vi "Periodic Tasks.vi"(8 "error in":errorcluster) -> ()   [LabVIEW 2020]
doc: "This VI runs in parallel to other tasks. It can contain as many user-defined periodic loops as you need. These can carry out PID or other sorts of timed response."
uses:
  <vilib>/Rock Robotics/WPI/ThirdParty/Phoenix-LabVIEW/Motor Controller/Controls/CTRE_Phoenix_MotorControl_ControlMode.ctl
  V1_nauru_2023_06_22/Global 1.vi
  <vilib>/Rock Robotics/Network Tables/NT Read Number.vi
  <vilib>/Rock Robotics/Network Tables/NT Write Number.vi
  <vilib>/Rock Robotics/WPI/Utilities/WPI_GetSetVariantRefNum.vi
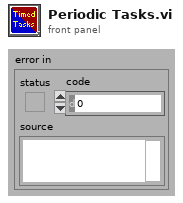
[diagram p1: front panel]
types:
  T1 = typedef "CTRE_Phoenix_MotorControl_ControlMode.ctl" = u16
  T2 = typedef "WPI_SwitchDevRef.ctl" = cluster{"DevStatus":errorcluster, "DIO Channel":T3, "CntIndex":T4, "Normally Closed":bool}
  T3 = typedef "FPGA_DIOChannel.ctl" = enum8{"DIO 0", "DIO 1", "DIO 2", "DIO 3", "DIO 4", "DIO 5", "DIO 6", "DIO 7", "DIO 8", "DIO 9", "DIO MXP 0", "DIO MXP 1", "DIO MXP 2", "DIO MXP 3", "DIO MXP 4", "DIO MXP 5", "DIO MXP 6", "DIO MXP 7", "DIO MXP 8", "DIO MXP 9", "DIO MXP 10", "DIO MXP 11", "DIO MXP 12", "DIO MXP 13", "DIO MXP 14", "DIO MXP 15", "SPI Port CS1", "SPI Port CS2", "SPI Port CS3", "SPI Port MISO", "SPI Port MOSI", "Invalid"}
  T4 = typedef "FPGA_CounterCtrSystemIndex.ctl" = enum8{"Ctr 0", "Ctr 1", "Ctr 2", "Ctr 3", "Ctr 4", "Ctr 5", "Ctr 6", "Ctr 7", "Invalid"}
  T5 = cluster{"Yaw":dbl, "Roll":dbl, "Pitch":dbl, "Heading":dbl, "Fused Heading":dbl}
  T6 = typedef "WPI_MotorControlDeviceRef.ctl" = cluster{"DeviceStatus":errorcluster, "Type":T7, "PWM":cluster{"PWM Channel":T8, "DeadBand":T9}, "CAN":cluster{"Device Number":u8, "SetOutput VI Ref":variant, "GetOutput VI Ref":variant, "Enable VI Ref":variant, "Disable VI Ref":variant, "Data":variant}, "Invert":bool, "DIO PWM":cluster{"PWM \"Enable\" Channel":T8, "DIOChannel":T3, "PWM Rate":dbl}}
  T7 = typedef "WPI_MotorControlType.ctl" = enum16{"PWM", "CAN", "DIO PWM"}
  T8 = typedef "FPGA_DIOPWMChannel.ctl" = enum8{"PWM 0", "PWM 1", "PWM 2", "PWM 3", "PWM 4", "PWM 5", "PWM 6", "PWM 7", "PWM 8", "PWM 9", "PWM MXP 0", "PWM MXP 1", "PWM MXP 2", "PWM MXP 3", "PWM MXP 4", "PWM MXP 5", "PWM MXP 6", "PWM MXP 7", "PWM MXP 8", "PWM MXP 9", "Invalid"}
  T9 = typedef "WPI_PWMDeadband.ctl" = cluster{"Name":string, "maxPositivePwm":i32, "minPositivePwm":i32, "centerPwm":i32, "maxNegativePwm":i32, "minNegativePwm":i32, "angularRange":u16}
  T10 = typedef "WPI_RobotDriveDevRef.ctl" = cluster{"DevStatus":errorcluster, "Motors[]":T6[], "Square Inputs":bool, "Max Output":dbl}
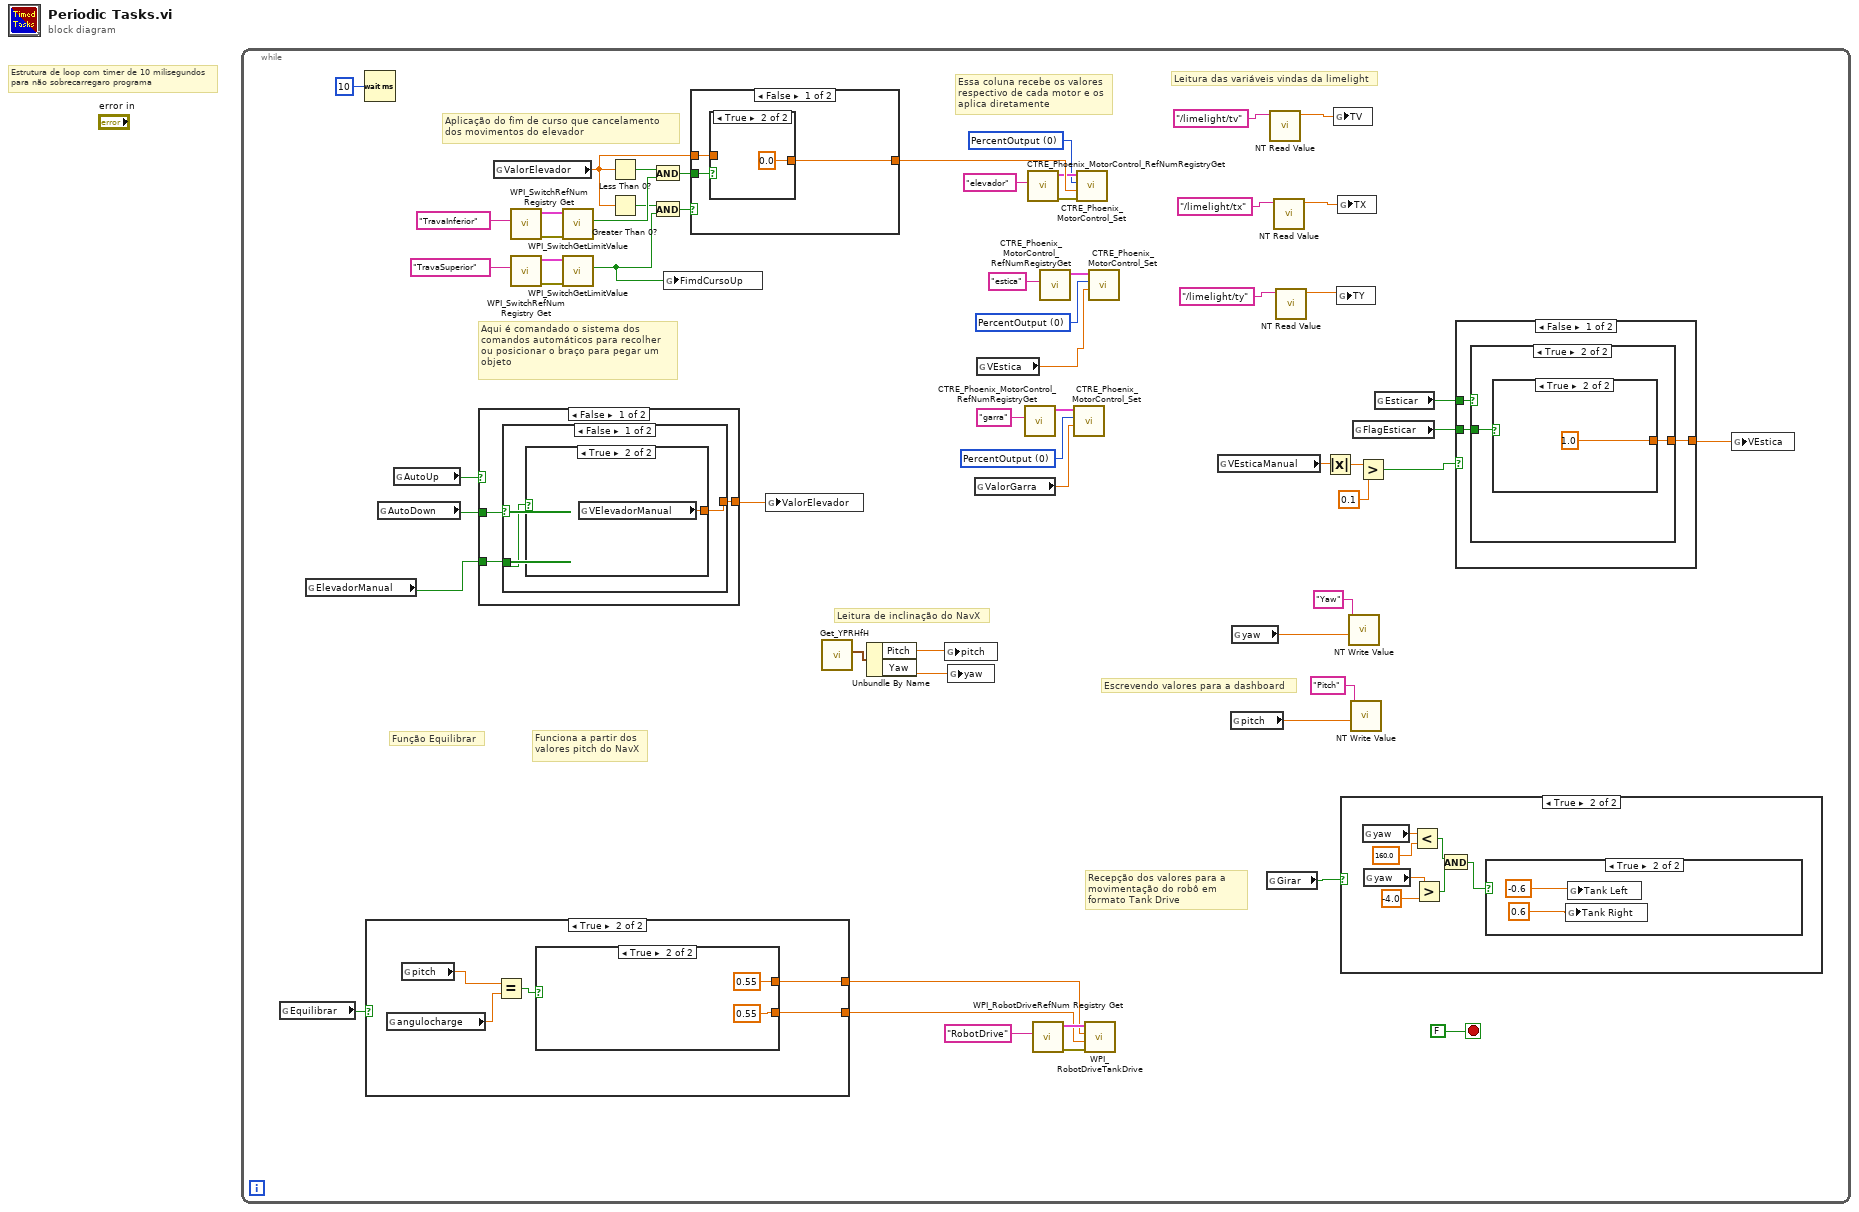
[diagram p0: block diagram]
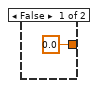
[diagram p2: hidden frame]
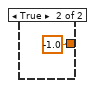
[diagram p3: hidden frame]
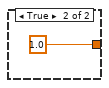
[diagram p4: hidden frame]
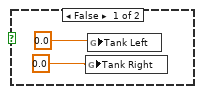
[diagram p6: hidden frame]
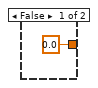
[diagram p7: hidden frame]
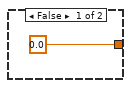
[diagram p8: hidden frame]
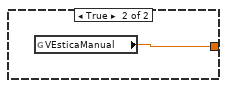
[diagram p9: hidden frame]
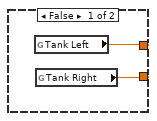
[diagram p10: hidden frame]
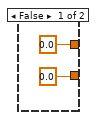
[diagram p11: hidden frame]
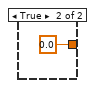
[diagram p13: hidden frame]
diagram:
  # "Estrutura de loop com timer de 10 milisegundos para não sobrecarregaro programa"
  n1 = while {
    stop <- FALSE stop-if-true
    w14 = T1 0 items=["PercentOutput"=0, "Position"=1, "Velocity"=2, "Current"=3, "Follower"=5, "MotionProfile"=6, "MotionMagic"=7, "MotionProfileArc"=10, "Disabled"=15] ("Control Mode")
    w36 = T1 0 items=["PercentOutput"=0, "Position"=1, "Velocity"=2, "Current"=3, "Follower"=5, "MotionProfile"=6, "MotionMagic"=7, "MotionProfileArc"=10, "Disabled"=15] ("Control Mode")
    w50 = T1 0 items=["PercentOutput"=0, "Position"=1, "Velocity"=2, "Current"=3, "Follower"=5, "MotionProfile"=6, "MotionMagic"=7, "MotionProfileArc"=10, "Disabled"=15] ("Control Mode")
    # "Escrevendo valores para a dashboard"
    # "Funciona a partir dos valores pitch do NavX"
    # "Função Equilibrar"
    # "Leitura de inclinação do NavX"
    # "Leitura das variáveis vindas da limelight"
    # "Recepção dos valores para a movimentação do robô em formato Tank Drive"
    # "Aplicação do fim de curso que cancelamento dos movimentos do elevador"
    # "Aqui é comandado o sistema dos comandos automáticos para recolher ou posicionar o braço para pegar um objeto"
    # "Essa coluna recebe os valores\nrespectivo de cada motor e os\naplica diretamente"
    n2 = global read "Global 1.vi" "Equilibrar"() -> (w27:bool)
    n3 = global read "Global 1.vi" "ElevadorManual"() -> (w2:bool)
    n4 = Wait (ms)(milliseconds to wait=u32 10) -> ()  [unwired: 1 out]
    n5 = case shown="True" w27 {
      tunnel: [w90 w91] -> w25
      tunnel: [w89 w92] -> w24
      frame False {
        n6 = global read "Global 1.vi" "Tank Left"() -> (w90:dbl)
        n7 = global read "Global 1.vi" "Tank Right"() -> (w89:dbl)
      }
      frame True {
        n8 = global read "Global 1.vi" "angulocharge"() -> (w94:dbl)
        n9 = global read "Global 1.vi" "pitch"() -> (w95:dbl)
        n10 = Equal?(x=w95, y=w94) -> (x = y?=w93:bool)
        n11 = case shown="True" w93 {
          tunnel: [0.0 ("Tank Right") 0.55 ("Tank Right")] -> w92
          tunnel: [0.0 ("Tank Left") 0.55 ("Tank Left")] -> w91
          frame False {
          }
          frame True {
          }
        }
      }
    }
    n12 = global read "Global 1.vi" "AutoDown"() -> (w3:bool)
    n13 = global read "Global 1.vi" "AutoUp"() -> (w4:bool)
    n14 = case shown="False" w4 {
      tunnel: w3 -> [w62 _]
      tunnel: [w61 1.0] -> w1
      tunnel: w2 -> [w60 _]
      frame False {
        n15 = case shown="False" w62 {
          tunnel: [w63 -1.0] -> w61
          tunnel: w60 -> [w64 _]
          frame False {
            n16 = case shown="True" w64 {
              tunnel: [0.0 ("ValorElevador") w66] -> w63
              frame False {
              }
              frame True {
                n17 = global read "Global 1.vi" "VElevadorManual"() -> (w66:dbl)
              }
            }
          }
          frame True {
          }
        }
      }
      frame True {
      }
    }
    n18 = global read "Global 1.vi" "ValorElevador"() -> (w39:dbl)
    n19 = call <vilib>:"WPI_SwitchRefNum Registry Get.vi"("refnum name"="TravaInferior") -> ("error out"=w46:errorcluster, "SwitchDevRef"=w45:T2)  [unwired: 9 in]
    n20 = call <vilib>:"WPI_SwitchRefNum Registry Get.vi"("refnum name"="TravaSuperior") -> ("error out"=w49:errorcluster, "SwitchDevRef"=w48:T2)  [unwired: 9 in]
    n21 = call <vilib>:"WPI_SwitchGetLimitValue.vi"("error in (no error)"=w46, "SwitchDevRef"=w45) -> ("Switch Pressed"=w54:bool)  [unwired: 7 in, 2 out]
    n22 = call <vilib>:"WPI_SwitchGetLimitValue.vi"("error in (no error)"=w49, "SwitchDevRef"=w48) -> ("Switch Pressed"=w34:bool)  [unwired: 7 in, 2 out]
    n23 = Less Than 0?(x=w39) -> (x < 0?=w42:bool)
    n24 = Greater Than 0?(x=w39) -> (x > 0?=w40:bool)
    n25 = And(x=w42, y=w54) -> (x .and. y?=w41:bool)
    n26 = And(x=w40, y=w34) -> (x .and. y?=w43:bool)
    n27 = global write "Global 1.vi" "FimdCursoUp"(w34) -> ()
    n28 = case shown="False" w43 {
      tunnel: [w101 0.0 ("Output")] -> w55
      tunnel: w41 -> [w102 _]
      tunnel: w39 -> [w100 _]
      frame False {
        n29 = case shown="True" w102 {
          tunnel: [w103 0.0 ("Output")] -> w101
          tunnel: w100 -> [w103 _]
          frame False {
          }
          frame True {
          }
        }
      }
      frame True {
      }
    }
    n30 = global write "Global 1.vi" "ValorElevador"(w1) -> ()
    n31 = call <vilib>:"Get_YPRHfH.vi"() -> ("YRPHfH"=w26:T5)  [unwired: 11 in]
    n32 = Unbundle By Name(w26) -> ("Pitch"=w10:dbl, "Yaw"=w9:dbl)
    n33 = global write "Global 1.vi" "pitch"(w10) -> ()
    n34 = global write "Global 1.vi" "yaw"(w9) -> ()
    n35 = global read "Global 1.vi" "ValorGarra"() -> (w35:dbl)
    n36 = global read "Global 1.vi" "VEstica"() -> (w13:dbl)
    n37 = call <vilib>:"CTRE_Phoenix_MotorControl_RefNumRegistryGet.vi"("refnum name"="garra") -> ("PhoenixMotorControlDevRef"=w38:T6)  [unwired: 9 in, 1 out]
    n38 = call <vilib>:"CTRE_Phoenix_MotorControl_RefNumRegistryGet.vi"("refnum name"="elevador") -> ("error out"=w53:errorcluster, "PhoenixMotorControlDevRef"=w52:T6)  [unwired: 9 in]
    n39 = call <vilib>:"WPI_RobotDriveRefNum Registry Get.vi"("refnum name"="RobotDrive") -> ("error out"=w57:errorcluster, "RobotDriveDevRef"=w58:T10)  [unwired: 9 in]
    n40 = call <vilib>:"CTRE_Phoenix_MotorControl_RefNumRegistryGet.vi"("refnum name"="estica") -> ("PhoenixMotorControlDevRef"=w16:T6)  [unwired: 9 in, 1 out]
    n41 = call <vilib>:"CTRE_Phoenix_MotorControl_Set.vi"("Output"=w35, "Control Mode"=w36, "PhoenixMotorControlDevRef"=w38) -> ()  [unwired: 7 in, 2 out]
    n42 = call <vilib>:"CTRE_Phoenix_MotorControl_Set.vi"("error in (no error)"=w53, "Output"=w55, "Control Mode"=w50, "PhoenixMotorControlDevRef"=w52) -> ()  [unwired: 6 in, 2 out]
    n43 = call <vilib>:"WPI_RobotDriveTankDrive.vi"("error in (no error)"=w57, "Right axis value"=w24, "Left axis value"=w25, "RobotDriveDevRef"=w58) -> ()  [unwired: 5 in, 3 out]
    n44 = call <vilib>:"CTRE_Phoenix_MotorControl_Set.vi"("Output"=w13, "Control Mode"=w14, "PhoenixMotorControlDevRef"=w16) -> ()  [unwired: 7 in, 2 out]
    n45 = global read "Global 1.vi" "VEsticaManual"() -> (w17:dbl)
    n46 = global read "Global 1.vi" "pitch"() -> (w6:dbl)
    n47 = global read "Global 1.vi" "yaw"() -> (w8:dbl)
    n48 = global read "Global 1.vi" "Girar"() -> (w11:bool)
    n49 = call-poly <vilib>:"NT Read Value.vi"("name"="/limelight/tv") -> ("value"=w28:dbl)  [unwired: 8 in, 2 out]
    n50 = call-poly <vilib>:"NT Read Value.vi"("name"="/limelight/tx") -> ("value"=w31:dbl)  [unwired: 8 in, 2 out]
    n51 = call-poly <vilib>:"NT Read Value.vi"("name"="/limelight/ty") -> ("value"=w30:dbl)  [unwired: 8 in, 2 out]
    n52 = Absolute Value(x=w17) -> (abs(x)=w20:dbl)
    n53 = global write "Global 1.vi" "TV"(w28) -> ()
    n54 = global write "Global 1.vi" "TY"(w30) -> ()
    n55 = global write "Global 1.vi" "TX"(w31) -> ()
    n56 = case shown="True" w11 {
      frame False {
      }
      frame True {
        n57 = global read "Global 1.vi" "yaw"() -> (w72:dbl)
        n58 = global read "Global 1.vi" "yaw"() -> (w74:dbl)
        n59 = Less?(x=w72, y=160.0) -> (x < y?=w73:bool)
        n60 = Greater?(x=w74, y=-4.0) -> (0:w75:bool)
        n61 = And(x=w73, y=w75) -> (x .and. y?=w69:bool)
        n62 = case shown="True" w69 {
          frame False {
            n63 = global write "Global 1.vi" "Tank Right"(0.0 ("Tank Left")) -> ()
            n64 = global write "Global 1.vi" "Tank Left"(0.0 ("Tank Left")) -> ()
          }
          frame True {
            n65 = global write "Global 1.vi" "Tank Right"(0.6 ("Tank Left")) -> ()
            n66 = global write "Global 1.vi" "Tank Left"(-0.6 ("Tank Left")) -> ()
          }
        }
      }
    }
    n67 = call-poly <vilib>:"NT Write Value.vi"("value"=w8, "name"="Yaw") -> ()  [unwired: 9 in, 1 out]
    n68 = call-poly <vilib>:"NT Write Value.vi"("value"=w6, "name"="Pitch") -> ()  [unwired: 9 in, 1 out]
    n69 = global read "Global 1.vi" "FlagEsticar"() -> (w12:bool)
    n70 = Greater?(x=w20, y=0.1) -> (0:w18:bool)
    n71 = global read "Global 1.vi" "Esticar"() -> (w21:bool)
    n72 = case shown="False" w18 {
      tunnel: w21 -> [w82 _]
      tunnel: [w81 w88] -> w22
      tunnel: w12 -> [w80 _]
      frame False {
        n73 = case shown="True" w82 {
          tunnel: [0.0 w85] -> w81
          tunnel: w80 -> [_ w84]
          frame False {
          }
          frame True {
            n74 = case shown="True" w84 {
              tunnel: [0.0 1.0] -> w85
              frame False {
              }
              frame True {
              }
            }
          }
        }
      }
      frame True {
        n75 = global read "Global 1.vi" "VEsticaManual"() -> (w88:dbl)
      }
    }
    n76 = global write "Global 1.vi" "VEstica"(w22) -> ()
  }
